vi "PM_test_elbow.vi"() -> ()   [LabVIEW 2014]
uses:
  <vilib>/rvi/Analysis/host/Butterworth/config/Butterworth Filter Order.ctl
  <vilib>/rvi/Analysis/host/Butterworth/config/Butterworth Filter Type.ctl
  <vilib>/FPGAPlugInAG/cRIO-9066/niLvFpga_Close_cRIO-9066.vi
  <vilib>/rvi/errors/niLvFpgaAdjustHostInterfaceError.vi
  <vilib>/Utility/error.llb/Error Cluster From Error Code.vi
  <vilib>/rvi/Analysis/host/Butterworth/config/BwScaledCoefficients.vi
  <vilib>/FPGAPlugInAG/cRIO-9066/niLvFpga_Open_cRIO-9066.vi
  <vilib>/rvi/interface/nirviCloseFPGA/nirviCloseFPGA.xnode
  FPGA Bitfiles/forcecontroledu_FPGATarget_impElbow_wp9Tcc+MyeY.lvbitx
  FPGA VIs/imp_Elbow.vi
  <vilib>/rvi/interface/nirviReadWriteControl/nirviReadWriteControl.xnode
  <vilib>/rvi/Analysis/host/Butterworth/XNode/ButterworthCoefficients.xnode
  <vilib>/rvi/interface/nirviOpenFPGA/nirviOpenFPGA.xnode
  <vilib>/rvi/Analysis/host/Public/NI_FpgaMspHost.lvlib
  NiFpgaLv.dll
panel:
  in  "cutoff frequency (Hz)_Dbtd":dbl=1000.0
  in  "cutoff frequency (Hz)_Dbtdd":dbl=1000.0
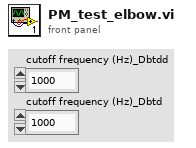
[diagram p1: front panel]
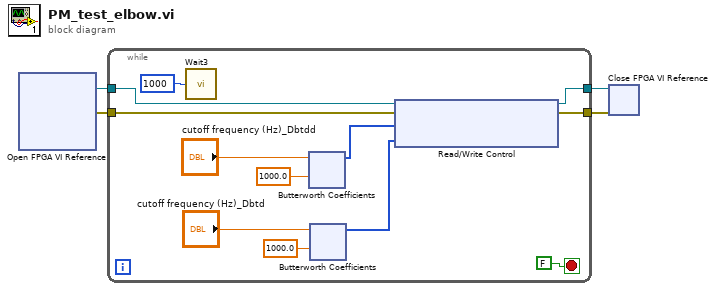
[diagram p0: block diagram]
diagram:
  n1 = xnode "Open FPGA VI Reference"() -> ("FPGA VI Reference Out"=w4:refnum<k20>, "error out"=w3:errorcluster)  [unwired: 2 in]
  n2 = while {
    tunnel: w4 -> [w13]
    tunnel: w3 -> [w12]
    tunnel: [w11] -> w2
    tunnel: [w10] -> w1
    stop <- FALSE stop-if-true
    n3 = call "Wait3"("Count(uSec)"=u32 1000 ("Count(mSec)")) -> ()  [unwired: 1 out]
    n4 = xnode "Butterworth Coefficients"("cutoff frequency (Hz)"="cutoff frequency (Hz)_Dbtdd", "sample rate (S/s)"=1000.0 ("sample rate (S/s)_Dytdd")) -> ("scaled coefficients"=w6:i32[])  [unwired: 1 in, 1 out]
    n5 = xnode "Butterworth Coefficients"("cutoff frequency (Hz)"="cutoff frequency (Hz)_Dbtd", "sample rate (S/s)"=1000.0 ("sample rate (S/s)_Dytd")) -> ("scaled coefficients"=w5:i32[])  [unwired: 1 in, 1 out]
    n6 = xnode "Read/Write Control"("FPGA VI Reference In"=w13, "error in"=w12, "scaled coefficients_Dbtdd"=w6, "scaled coefficients_Dbtd"=w5) -> ("FPGA VI Reference Out"=w11:refnum<k20>, "error out"=w10:errorcluster)
  }
  n7 = xnode "Close FPGA VI Reference"("FPGA VI Reference In"=w2, "error in"=w1) -> ()  [unwired: 1 out]
